vi "Get Supported Targets.vi"(8 "error in":errorcluster, 11 "user tag bus module configuration In":refnum<class "TEST CONFIGURATION.lvclass">) -> (0 "error out":errorcluster, 2 "supported targets":T1[](array[typedef]), 3 "user tag bus module configuration Out":refnum<class "TEST CONFIGURATION.lvclass">)   [LabVIEW 2013, in "configuration tests.lvlib" / "TEST CONFIGURATION.lvclass"]
doc: "Provides an interface for determining the targets supported by a given module configuration/runtime class pairing. This should be overridden by any useful child class."
uses:
  TEST CONFIGURATION.lvclass
  <vilib>/NI/Tag Bus Module Framework/root configuration/Target Types.ctl
  <vilib>/NI/Tag Bus Module Framework/root configuration/TBM configuration.lvclass
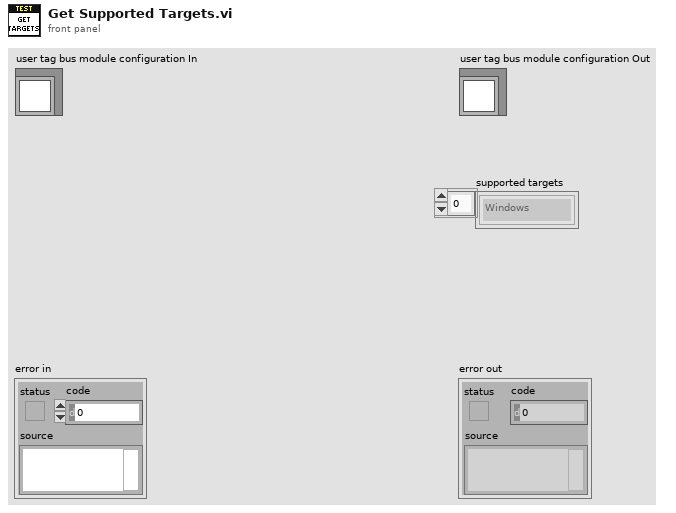
[diagram p1: front panel]
types:
  T1 = typedef "TBM configuration.lvclass/Target Types.ctl" = enum16{"Windows", "Mac", "Linux", "Linux RT ARM", "VxWorks", "Pharlap", "Other", "Linux RT x64"}
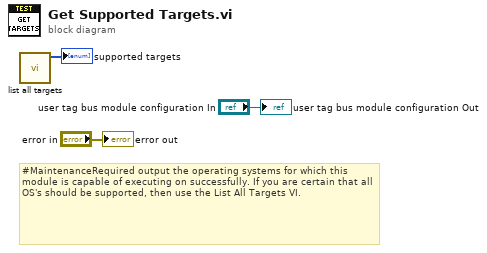
[diagram p0: block diagram]
diagram:
  # "#MaintenanceRequired output the operating systems for which this module is capable of executing on successfully. If you are certain that all OS's should be supported, then use the List All Targets VI."
  n1 = call <vilib>:"list all targets.vi"() -> ("all targets"=→"supported targets":T1[])  [unwired: 11 in]
  "error out" <- "error in"
  "user tag bus module configuration Out" <- "user tag bus module configuration In"
